vi "Load-Defaults.vi"(8 "error in (no error)":errorcluster, 9 "VI path":path, 11 "configuration file path":path) -> (0 "error out":errorcluster)   [LabVIEW 2020, in "Save-Load-Defaults.lvlib"]
doc: "This VI loads the values of the controls of the VI specified in VI path from settings.dat using the Configuration File VIs."
uses:
  Save-Load-Defaults.lvlib
  <vilib>/Utility/config.llb/Read Key (String).vi
  <vilib>/Utility/config.llb/NI_LVConfig.lvlib
panel:
  # "Load Default Values - fill in file-paths to automatically load previously\nsaved control values."
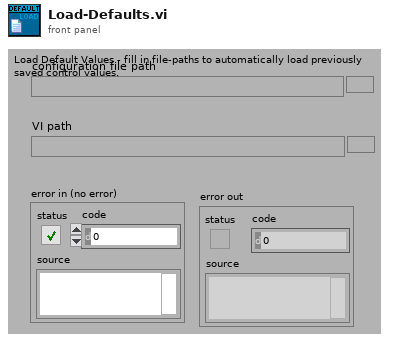
[diagram p1: front panel]
types:
  T1 = typedef "NI_LVConfig.lvlib/Config Data RefNum.ctl" = refnum<k1>
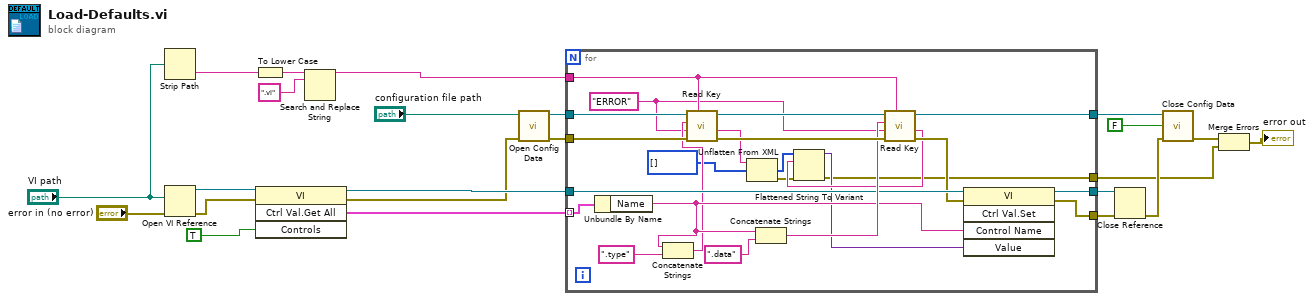
[diagram p0: block diagram]
diagram:
  n1 = Strip Path(path="VI path") -> (name=w14:string)  [unwired: 1 out]
  n2 = Open VI Reference(vi path="VI path", error in (no error)="error in (no error)") -> (vi reference=w9:refnum<vi>, error out=w11:errorcluster)  [unwired: 4 in]
  n3 = To Lower Case(string=w14) -> (all lower case string=w15:string)
  n4 = invoke class="VI" method="Ctrl Val.Get All"(reference=w9, error in=w11, "Controls"=TRUE ("controls")) -> (reference out=w21:refnum<vi>, error out=w8:errorcluster, "Get All Control Values Variant"=w22:cluster{"Name":string, "Variant Data":variant}[])  [unwired: 1 in, 1 out]
  n5 = Search and Replace String(input string=w15, search string=".vi") -> (result string=w23:string)  [unwired: 6 in, 3 out]
  n6 = call <vilib>:"Open Config Data.vi"("error in (no error)"=w8, "configuration file path"="configuration file path") -> ("error out"=w5:errorcluster, "refnum"=w6:T1)  [unwired: 7 in, 1 out]
  n7 = for {
    tunnel: w22 -> [w47] mode=indexing
    tunnel: w23 -> [w40]
    tunnel: w21 -> [w38]
    tunnel: w5 -> [w45]
    tunnel: w6 -> [w46]
    tunnel: [w33] -> w20
    tunnel: [w32] -> w18
    tunnel: [w31] -> w17
    tunnel: [w24] -> w1
    w35 = "ERROR" ("section")
    n8 = Unbundle By Name(w47) -> ("Name"=w37:string)
    n9 = Concatenate Strings(w37, ".type" ("string")) -> (w36:string)
    n10 = call-poly <vilib>:"Read Key.vi"("section"=w40, "error in (no error)"=w45, "default value"=w35, "key"=w36, "refnum"=w46) -> ("error out"=w41:errorcluster, "value"=w28:string, "refnum out"=w42:T1)  [unwired: 3 in, 1 out]
    n11 = Unflatten From XML(xml string=w28, type=i16[] [] ("Array")) -> (value=w27:i16[], error out=w25:errorcluster)  [unwired: 1 in]
    n12 = Concatenate Strings(w37, ".data" ("string")) -> (w39:string)
    n13 = call-poly <vilib>:"Read Key.vi"("section"=w40, "error in (no error)"=w41, "default value"=w35, "key"=w39, "refnum"=w42) -> ("error out"=w34:errorcluster, "value"=w30:string, "refnum out"=w33:T1)  [unwired: 3 in, 1 out]
    n14 = Flattened String To Variant(4:w25, 6:w30, 7:w27) -> (0:w24:errorcluster, 3:w26:variant)
    n15 = invoke class="VI" method="Ctrl Val.Set"(reference=w38, error in=w34, "Control Name"=w37, "Value"=w26) -> (reference out=w32:refnum<vi>, error out=w31:errorcluster)  [unwired: 1 in, 3 out]
  }
  n16 = Close Reference(reference=w18, error in (no error)=w17) -> (error out=w16:errorcluster)
  n17 = call <vilib>:"Close Config Data.vi"("error in (no error)"=w16, "write file if changed (T)"=FALSE ("write configuration file? (T)"), "refnum"=w20) -> ("error out"=w3:errorcluster)  [unwired: 7 in, 1 out]
  n18 = Merge Errors(w3, w1) -> (→"error out":errorcluster)
